vi "Z Aux Direct M Helical.vi"(0 "handle":u32, 1 "fcenter2":sgl, 2 "fDistance3":sgl, 5 "fend1":sgl, 7 "fend2":sgl, 9 "fcenter1":sgl, 11 "error in (no error)":errorcluster caption="错误输入（无错误）", 12 "idirection":i32, 13 "imode":i32) -> (4 "handle out":u32, 6 "function return":i32, 15 "error out":errorcluster caption="错误输出")   [LabVIEW 2015, in "zauxdll.lvlib"]
doc: "int32 __stdcall ZAux_Direct_MHelical(ZMC_HANDLE handle, float fend1, float fend2, float fcenter1, float fcenter2, int idirection, float fDistance3, int imode);"
uses:
  zauxdll.lvlib
  Radar - 2015 32bit_autoqueue_angle_0319/zauxdll-2014/zauxdll.dll
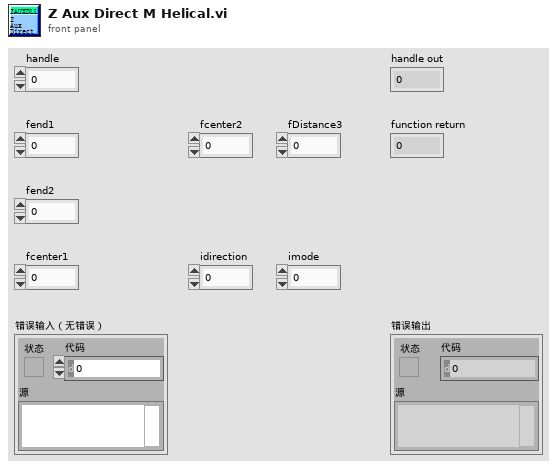
[diagram p1: front panel]
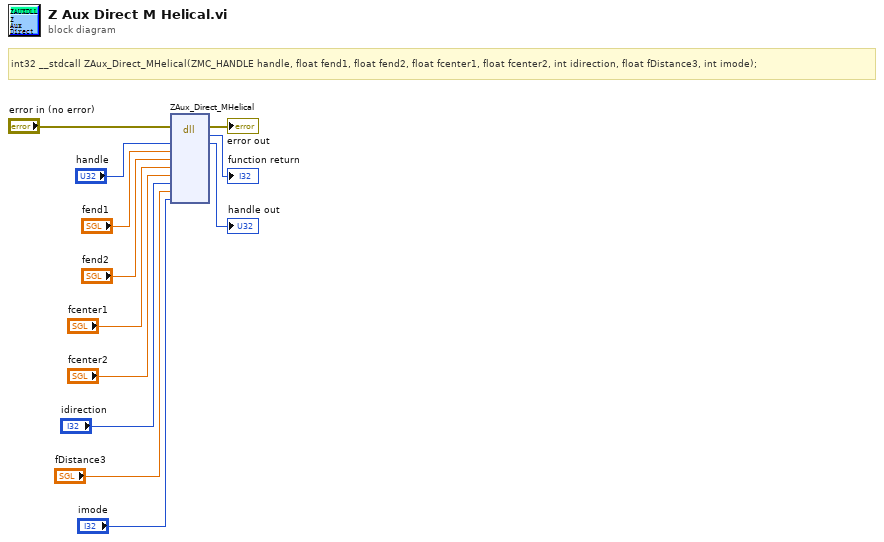
[diagram p0: block diagram]
diagram:
  # "int32 __stdcall ZAux_Direct_MHelical(ZMC_HANDLE handle, float fend1, float fend2, float fcenter1, float fcenter2, int idirection, float fDistance3, int imode);"
  n1 = dll-call lib="D:/vicomm case/cub/0717/Radar - 2015 32bit_autoqueue_angle_0319/zauxdll-2014/zauxdll.*" fn="ZAux_Direct_MHelical"(error in="error in (no error)", "handle"="handle", "fend1"="fend1", "fend2"="fend2", "fcenter1"="fcenter1", "fcenter2"="fcenter2", "idirection"="idirection", "fDistance3"="fDistance3", "imode"="imode") -> (error out=→"error out":errorcluster, →"function return":i32, "handle"=→"handle out":u32)  [unwired: 9 in, 1 out]
